vi "loopTest.vi"() -> ()   [LabVIEW 2022 SP3]
panel:
  in  "milliseconds to wait":u32=1000
  in  "Stop Button":bool
  out "XY Graph":T1(graph)
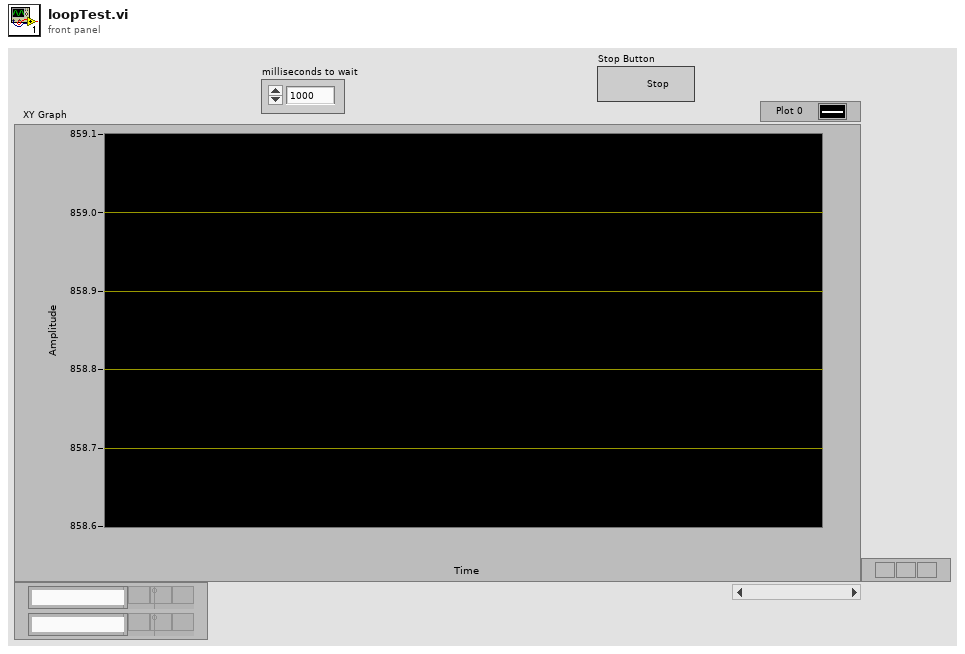
[diagram p1: front panel]
types:
  T1 = cluster{"seconds since 1Jan1904":timestamp, "Pressure(hPa)":dbl}[]
  T2 = cluster{"seconds since 1Jan1904":timestamp, "Pressure(hPa)":dbl}
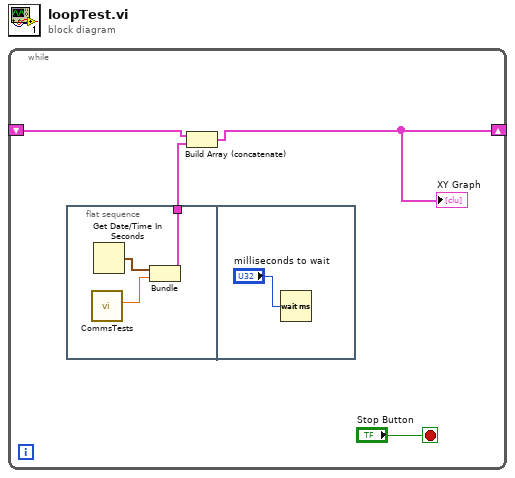
[diagram p0: block diagram]
diagram:
  n1 = while {
    shift-right: [w2] -> _
    shift-left: _ -> [w3]
    stop <- "Stop Button" stop-if-true
    n2 = flat-sequence {
      tunnel: [w5] -> w1
      frame #0 {
        n3 = call "CommsTests.vi"() -> ("Pressure(hPa)"=w6:dbl)  [unwired: 11 in]
        n4 = Get Date/Time In Seconds() -> (seconds since 1Jan1904=w7:timestamp)
        n5 = Bundle("seconds since 1Jan1904"=w7, "Pressure(hPa)"=w6) -> (w5:T2)  [unwired: 1 in]
      }
      frame #1 {
        n6 = Wait (ms)(milliseconds to wait="milliseconds to wait") -> ()  [unwired: 1 out]
      }
    }
    n7 = Build Array (concatenate)(w3, w1) -> (w2:T1)
    "XY Graph" <- w2
  }
